vi "2048_cal_row.vi"(10 "VKey":T1, 11 "Array in":i32[](array[numeric])) -> (2 "score_add":i32, 3 "Array out":i32[](array[numeric]))   [LabVIEW 2022 SP3]
uses:
  <vilib>/event_ctls.llb/eventvkey.ctl
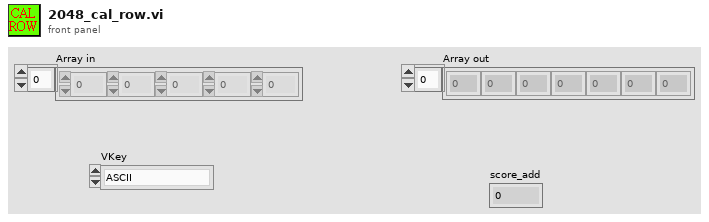
[diagram p1: front panel]
types:
  T1 = typedef "eventvkey.ctl" = enum16{"ASCII", "Enter", "Return", "Shift", "Ctrl", "Alt", "Cmd", "Opt", "Caps", "NumLock", "Clear", "Break", "Up", "Down", "Left", "Right", "Insert", "Delete", "Home", "End", "PageUp", "PageDown", "Escape", "Help", "Pause", "ScrollLock", "F1", "F2", "F3", "F4", "F5", "F6", "F7", "F8", "F9", "F10", "F11", "F12", "F13", "F14", "F15", "F16", "F17", "F18", "F19", "F20", "F21", "F22", "F23", "F24", "Play", "VolumeUp", "VolumeDown", "Mute", "Two Byte Char"}
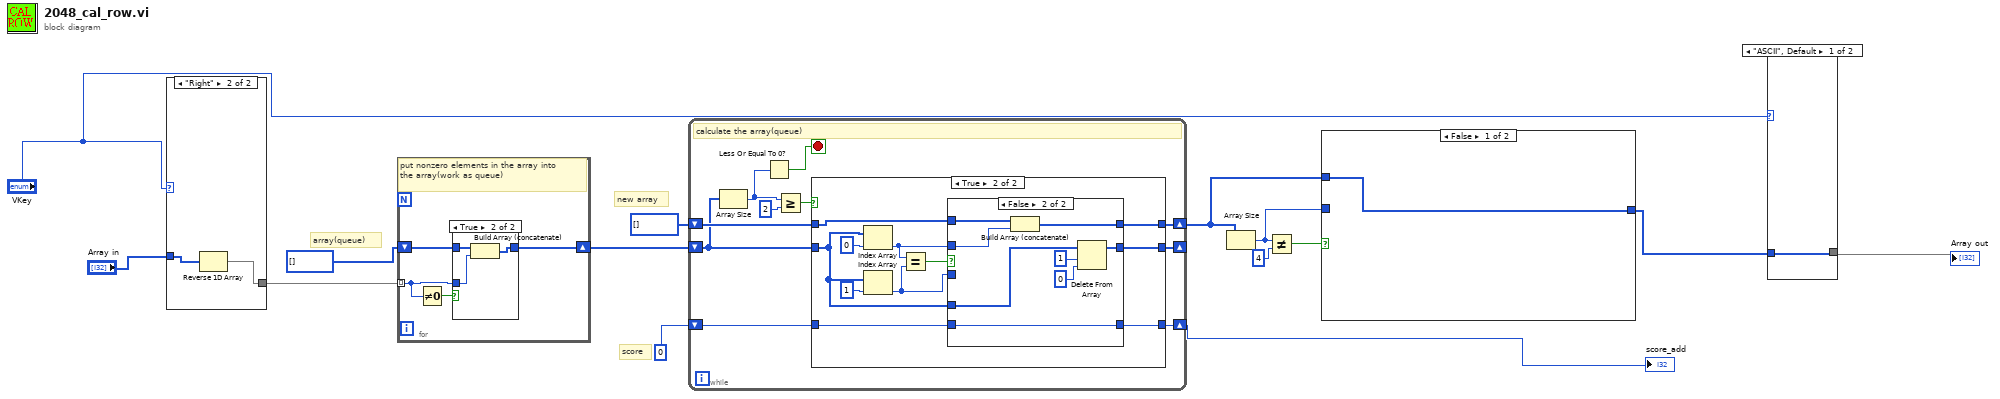
[diagram p0: block diagram]
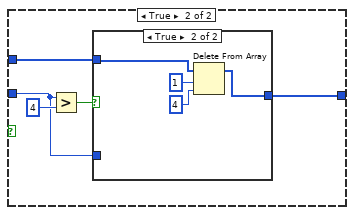
[diagram p2: hidden frame]
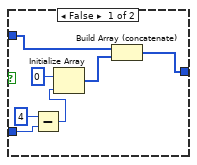
[diagram p3: hidden frame]
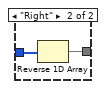
[diagram p4: hidden frame]
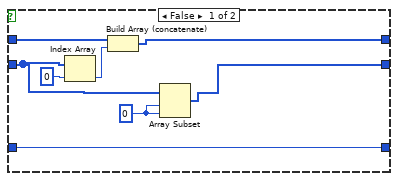
[diagram p6: hidden frame]
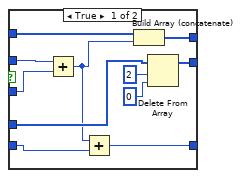
[diagram p7: hidden frame]
diagram:
  # "new array"
  # "score"
  # "array(queue)"
  n1 = case shown="\"Right\"" "VKey" {
    tunnel: "Array in" -> [w15 w17]
    tunnel: [w15 w16] -> w10
    frame "ASCII", Default {
    }
    frame "Right" {
      n2 = Reverse 1D Array(array=w17) -> (reversed array=w16:i32[])
    }
  }
  n3 = for {
    tunnel: w10 -> [w19] mode=indexing
    shift-right: [w18] -> w14
    shift-left: i32[] [] -> [w20]
    # "put nonzero elements in the array into the array(work as queue)"
    n4 = Not Equal To 0?(x=w19) -> (x != 0?=w21:bool)
    n5 = case shown="True" w21 {
      tunnel: w20 -> [w22 w25]
      tunnel: w19 -> [_ w24]
      tunnel: [w22 w23] -> w18
      frame False {
      }
      frame True {
        n6 = Build Array (concatenate)(w25, w24) -> (w23:i32[])
      }
    }
  }
  n7 = while {
    shift-right: [w30] -> _
    shift-left: w14 -> [w28]
    shift-right: [w31] -> w3
    shift-left: i32[] [] -> [w32]
    shift-right: [w26] -> w8
    shift-left: 0 -> [w27]
    stop <- w35 stop-if-true
    # "calculate the array(queue)"
    n8 = Array Size(array=w28) -> (size(s)=w29:i32)
    n9 = Less Or Equal To 0?(x=w29) -> (x <= 0?=w35:bool)
    n10 = Greater Or Equal?(x=w29, y=2) -> (x >= y?=w33:bool)
    n11 = case shown="True" w33 {
      tunnel: w32 -> [w43 w53]
      tunnel: [w39 w52] -> w31
      tunnel: [w37 w51] -> w30
      tunnel: w28 -> [w38 w46]
      tunnel: w27 -> [w40 w45]
      tunnel: [w40 w44] -> w26
      frame False {
        w36 = 0 ("length")
        n12 = Index Array(array=w38, index=0) -> (element=w41:i32)
        n13 = Build Array (concatenate)(w43, w41) -> (w39:i32[])
        n14 = Array Subset(array=w38, index=w36, length=w36) -> (w37:i32[])
      }
      frame True {
        n15 = Index Array(array=w46, index=0) -> (element=w48:i32)
        n16 = Index Array(array=w46, index=1) -> (element=w47:i32)
        n17 = Equal?(x=w48, y=w47) -> (x = y?=w54:bool)
        n18 = case shown="False" w54 {
          tunnel: w48 -> [w62 w71]
          tunnel: w53 -> [w65 w73]
          tunnel: [w64 w72] -> w52
          tunnel: [w58 w68] -> w51
          tunnel: w47 -> [w63 _]
          tunnel: w46 -> [w61 w67]
          tunnel: w45 -> [w57 w66]
          tunnel: [w55 w66] -> w44
          frame True {
            n19 = Add(x=w62, y=w63) -> (x+y=w56:i32)
            n20 = Add(x=w56, y=w57) -> (x+y=w55:i32)
            n21 = Build Array (concatenate)(w65, w56) -> (w64:i32[])
            n22 = Delete From Array(array=w61, length=2, index=0) -> (array with subset deleted=w58:i32[])  [unwired: 1 out]
          }
          frame False {
            n23 = Build Array (concatenate)(w73, w71) -> (w72:i32[])
            n24 = Delete From Array(array=w67, length=1, index=0) -> (array with subset deleted=w68:i32[])  [unwired: 1 out]
          }
        }
      }
    }
  }
  "score_add" <- w8
  n25 = Array Size(array=w3) -> (size(s)=w2:i32)
  n26 = Not Equal?(x=w2, y=4) -> (x != y?=w4:bool)
  n27 = case shown="False" w4 {
    tunnel: w3 -> [w74 w79]
    tunnel: [w74 w78] -> w1
    tunnel: w2 -> [_ w75]
    frame False {
    }
    frame True {
      n28 = Greater?(x=w75, y=4) -> (0:w77:bool)
      n29 = case shown="True" w77 {
        tunnel: w79 -> [w86 w90]
        tunnel: [w80 w87] -> w78
        tunnel: w75 -> [w83 _]
        frame False {
          n30 = Subtract(x=4, y=w83) -> (x-y=w82:i32)
          n31 = Initialize Array(0 ("element"), w82) -> (w81:i32[])
          n32 = Build Array (concatenate)(w86, w81) -> (w80:i32[])
        }
        frame True {
          n33 = Delete From Array(array=w90, length=1, index=4) -> (array with subset deleted=w87:i32[])  [unwired: 1 out]
        }
      }
    }
  }
  n34 = case shown="\"ASCII\", Default" "VKey" {
    tunnel: w1 -> [w91 w93]
    tunnel: [w91 w92] -> w6
    frame "ASCII", Default {
    }
    frame "Right" {
      n35 = Reverse 1D Array(array=w93) -> (reversed array=w92:i32[])
    }
  }
  "Array out" <- w6
